vi "EOL CAN_Start_Teach.vi"(7 "Rx Arbitration Id":u32=402522244 format="%.0x", 8 "Error in":errorcluster, 9 "Glass?":bool, 10 "Read Session in":refnum<k21>, 11 "Write Session in":refnum<k21>) -> (0 "Error out":errorcluster, 2 "TxRx Data":string[][](array[string]), 3 "Response Good?":bool)   [LabVIEW 2014]
uses:
  <vilib>/xnet/xnet.llb/XNET Frame CAN.ctl
  <vilib>/xnet/xnet.llb/XNET Frame Type CAN.ctl
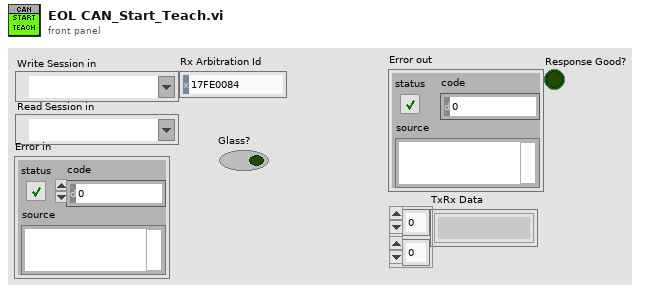
[diagram p1: front panel]
types:
  T1 = typedef "XNET Frame CAN.ctl" = cluster{"timestamp":timestamp, "payload":u8[], "identifier":u32, "type":T2, "extended?":bool, "echo?":bool}
  T2 = typedef "XNET Frame Type CAN.ctl" = u8
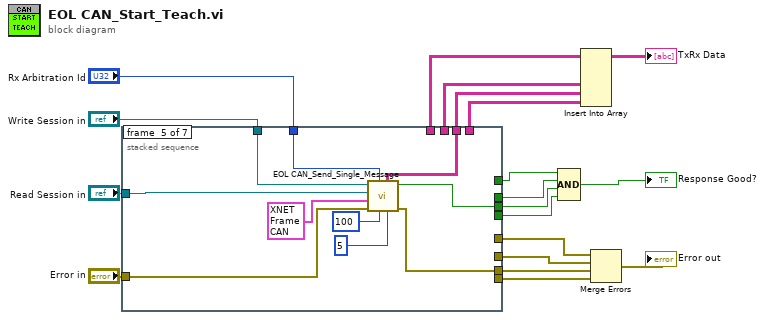
[diagram p0: block diagram]
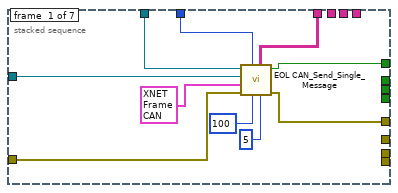
[diagram p2: hidden frame]
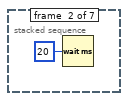
[diagram p3: hidden frame]
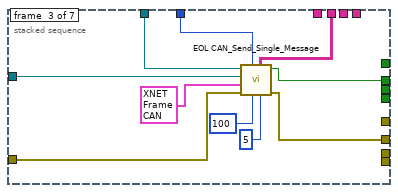
[diagram p4: hidden frame]
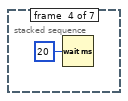
[diagram p5: hidden frame]
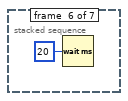
[diagram p6: hidden frame]
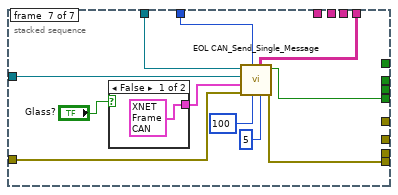
[diagram p7: hidden frame]
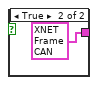
[diagram p8: hidden frame]
diagram:
  n1 = stacked-sequence {
    tunnel: [w29 _ _ _ _ _ _] -> w19
    tunnel: [w28 _ _ _ _ _ _] -> w9
    tunnel: [w24 _ _ _ _ _ _] -> w18
    tunnel: "Error in" -> [w20 _ w40 _ w48 _ w60]
    tunnel: "Read Session in" -> [w21 _ w39 _ w50 _ w56]
    tunnel: "Write Session in" -> [w22 _ w38 _ w49 _ w55]
    tunnel: "Rx Arbitration Id" -> [w23 _ w37 _ w43 _ w54]
    tunnel: [_ _ w36 _ _ _ _] -> w12
    tunnel: [_ _ w35 _ _ _ _] -> w10
    tunnel: [_ _ _ _ _ _ w59] -> w4
    tunnel: [_ _ _ _ _ _ w58] -> w2
    tunnel: [_ _ w34 _ _ _ _] -> w7
    tunnel: [_ _ _ _ _ _ w57] -> w6
    tunnel: [_ _ _ _ w45 _ _] -> w5
    tunnel: [_ _ _ _ w44 _ _] -> w3
    tunnel: [_ _ _ _ w42 _ _] -> w1
    frame #0 {
      n2 = call "EOL CAN_Send_Single_Message.vi"("Retries"=5, "Msg Wait Time"=u32 100, "Rx Arbitration Id"=w23, "Error in"=w20, "Tx CAN frame"=T1 {"timestamp"=timestamp(0 s since 1904-01-01), "payload"=[2, 16, 79, 85, 85, 85, 85, 85], "identifier"=402391172, "type"=8, "extended?"=TRUE, "echo?"=FALSE}, "Read Session in"=w21, "Write Session in"=w22) -> ("Error out"=w24:errorcluster, "Response Good?"=w28:bool, "TxRx Data"=w29:string[][])  [unwired: 2 out]
    }
    frame #1 {
      n3 = Wait (ms)(milliseconds to wait=u32 20) -> ()  [unwired: 1 out]
    }
    frame #2 {
      n4 = call "EOL CAN_Send_Single_Message.vi"("Retries"=5, "Msg Wait Time"=u32 100, "Rx Arbitration Id"=w37, "Error in"=w40, "Tx CAN frame"=T1 {"timestamp"=timestamp(0 s since 1904-01-01), "payload"=[2, 16, 64, 85, 85, 85, 85, 85], "identifier"=402391172, "type"=8, "extended?"=TRUE, "echo?"=FALSE}, "Read Session in"=w39, "Write Session in"=w38) -> ("Error out"=w34:errorcluster, "Response Good?"=w35:bool, "TxRx Data"=w36:string[][])  [unwired: 2 out]
    }
    frame #3 {
      n5 = Wait (ms)(milliseconds to wait=u32 20) -> ()  [unwired: 1 out]
    }
    frame #4 {
      n6 = call "EOL CAN_Send_Single_Message.vi"("Retries"=5, "Msg Wait Time"=u32 100, "Rx Arbitration Id"=w43, "Error in"=w48, "Tx CAN frame"=T1 {"timestamp"=timestamp(0 s since 1904-01-01), "payload"=[7, 49, 1, 5, 39, 64, 0, 0], "identifier"=402391172, "type"=8, "extended?"=TRUE, "echo?"=FALSE}, "Read Session in"=w50, "Write Session in"=w49) -> ("Error out"=w45:errorcluster, "Response Good?"=w44:bool, "TxRx Data"=w42:string[][])  [unwired: 2 out]
    }
    frame #5 {
      n7 = Wait (ms)(milliseconds to wait=u32 20) -> ()  [unwired: 1 out]
    }
    frame #6 {
      n8 = case shown="False" "Glass?" {
        tunnel: [T1 {"timestamp"=timestamp(0 s since 1904-01-01), "payload"=[7, 49, 1, 5, 36, 64, 0, 0], "identifier"=402391172, "type"=8, "extended?"=TRUE, "echo?"=FALSE} ("Tx CAN frame") T1 {"timestamp"=timestamp(0 s since 1904-01-01), "payload"=[7, 49, 1, 5, 35, 64, 0, 0], "identifier"=402391172, "type"=8, "extended?"=TRUE, "echo?"=FALSE} ("Tx CAN frame")] -> w61
        frame False {
        }
        frame True {
        }
      }
      n9 = call "EOL CAN_Send_Single_Message.vi"("Retries"=5, "Msg Wait Time"=u32 100, "Rx Arbitration Id"=w54, "Error in"=w60, "Tx CAN frame"=w61, "Read Session in"=w56, "Write Session in"=w55) -> ("Error out"=w57:errorcluster, "Response Good?"=w59:bool, "TxRx Data"=w58:string[][])  [unwired: 2 out]
    }
  }
  n10 = Compound Arithmetic op=AND(w9, w10, w3, w4) -> (→"Response Good?":bool)
  n11 = Insert Into Array(array=w19, new element #1=w12, new element #2=w1, new element #3=w2) -> (→"TxRx Data":string[][])  [unwired: 2 in]
  n12 = Merge Errors(w18, w7, w5, w6) -> (→"Error out":errorcluster)
